vi "front pannel.vi"() -> ()   [LabVIEW 2013]
uses:
  XPS-C8 Controller/Examples/Global 1.vi
panel:
  out "KILL ALL ERROR":string
  in  "KILL ALL":bool
  out "error status 8":string
  out "error status 7":string
  out "error status 6":string
  out "error status 5":string
  out "error status 4":string
  out "error status 3":string
  out "error status 2":string
  out "error status 1":string
  out "position 8":dbl format="%#_13g"
  out "position 7":dbl format="%#_13g"
  out "position 6":dbl format="%#_13g"
  out "position 5":dbl format="%#_13g"
  out "position 4":dbl format="%#_13g"
  out "position 3":dbl format="%#_13g"
  out "position 2":dbl format="%#_13g"
  out "position 1":dbl format="%#_13g"
  in  "move 8":bool
  in  "move 7":bool
  in  "move 6":bool
  in  "move 5":bool
  in  "move 4":bool
  in  "move 3":bool
  in  "move 2":bool
  in  "move 1":bool
  out "8":bool
  out "7":bool
  out "6":bool
  out "5":bool
  out "4":bool
  out "3":bool
  out "2":bool
  out "error":bool
  out "hardware status 8":string
  out "hardware status 7":string
  out "hardware status 6":string
  out "hardware status 5":string
  out "hardware status 4":string
  out "hardware status 3":string
  out "hardware status 2":string
  out "hardware status 1":string
  out "motor name 8":string
  out "motor name 7":string
  out "motor name 6":string
  out "motor name 5":string
  out "motor name 4":string
  out "motor name 3":string
  out "motor name 2":string
  out "motor name 1":string
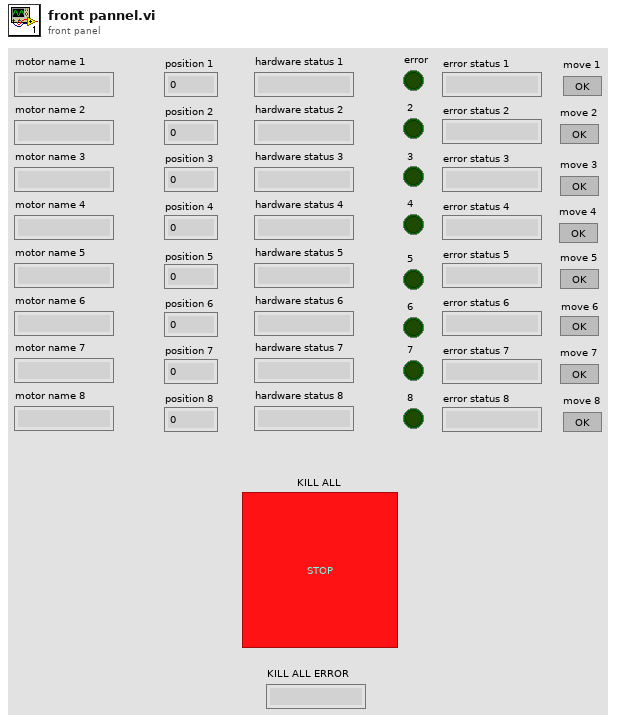
[diagram p1: front panel]
types:
  T1 = cluster{"connection TCP":refnum<k5>, "LogTo File":bool, "Log File refnum":refnum<file>, "no error if error log":bool}
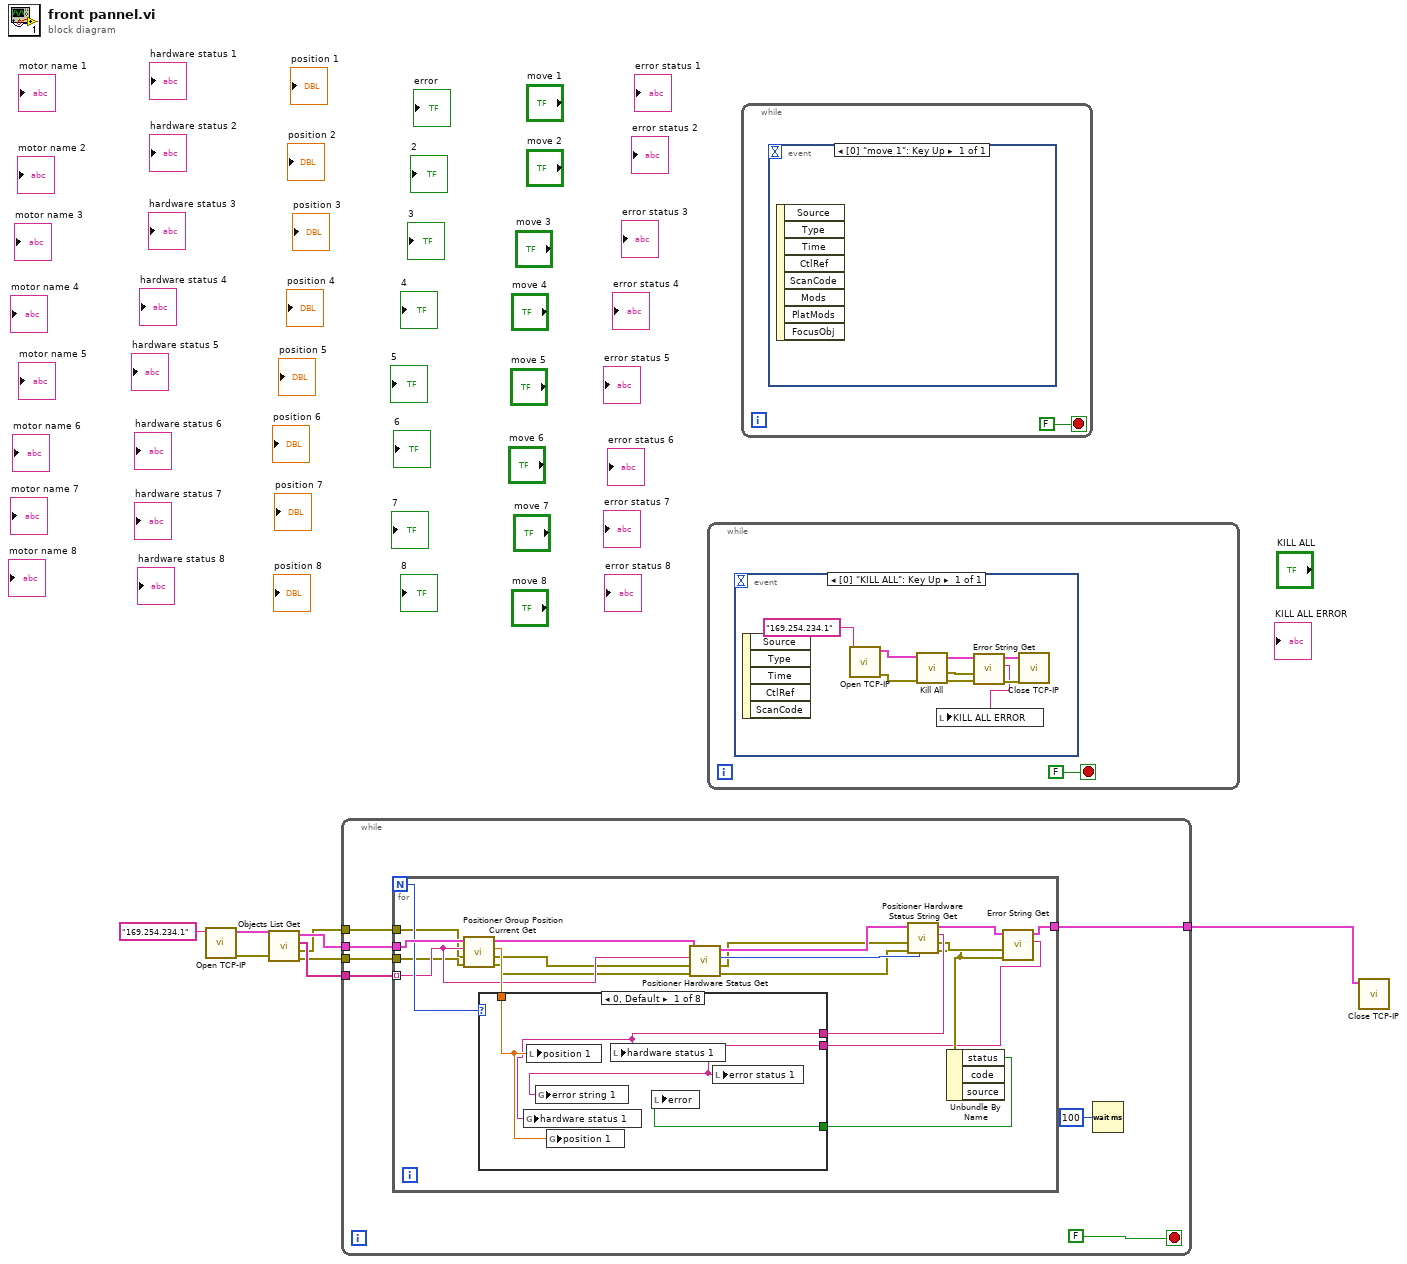
[diagram p0: block diagram]
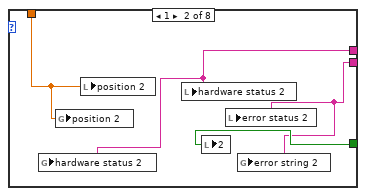
[diagram p2: hidden frame]
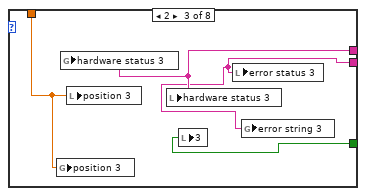
[diagram p3: hidden frame]
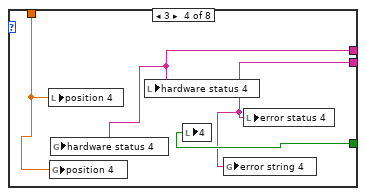
[diagram p4: hidden frame]
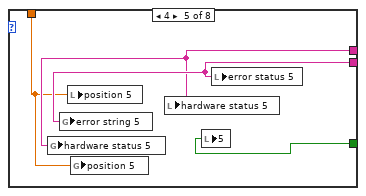
[diagram p5: hidden frame]
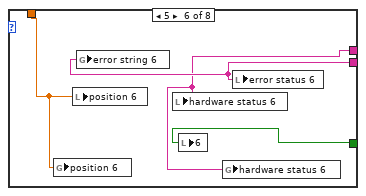
[diagram p6: hidden frame]
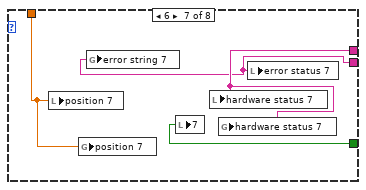
[diagram p7: hidden frame]
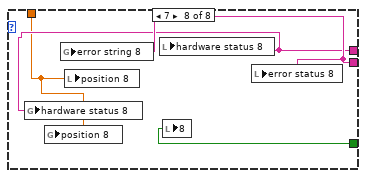
[diagram p8: hidden frame]
diagram:
  n1 = call <userlib>:"Open TCP-IP.vi"("IP address"="169.254.234.1") -> ("error out"=w3:errorcluster, "Connection ID"=w7:T1)  [unwired: 8 in, 1 out]
  n2 = call <userlib>:"Objects List Get.vi"("error in (no error)"=w3, "connection ID in"=w7) -> ("error out"=w2:errorcluster, "XPS error out"=w1:errorcluster, "Positioners"=w8:string[], "connection ID out"=w6:T1)  [unwired: 4 in, 2 out]
  n3 = while {
    tunnel: w8 -> [w15]
    tunnel: w6 -> [w14]
    tunnel: [w11] -> w5
    tunnel: w2 -> [w10]
    tunnel: w1 -> [w9]
    stop <- FALSE stop-if-true
    n4 = for {
      N -> [w31]
      tunnel: w15 -> [w28] mode=indexing
      tunnel: w14 -> [w35]
      tunnel: [w17] -> w11
      tunnel: w10 -> [w27]
      tunnel: w9 -> [w23]
      n5 = call "Positioner Group Position Current Get.vi"("error in (no error)"=w27, "XPS error in (no error)"=w23, "Positioner Name (250 c max)"=w28, "connection ID in"=w35) -> ("error out"=w26:errorcluster, "XPS error out"=w22:errorcluster, "Current position (units)"=w30:dbl, "connection ID out"=w34:T1)  [unwired: 4 in]
      n6 = call "Positioner Hardware Status Get.vi"("error in (no error)"=w26, "XPS error in (no error)"=w22, "Positioner Name (250 c max)"=w28, "connection ID in"=w34) -> ("error out"=w25:errorcluster, "XPS error out"=w21:errorcluster, "Positioner Hardware Status"=w32:i32, "connection ID out"=w33:T1)  [unwired: 4 in]
      n7 = call "Positioner Hardware Status String Get.vi"("Positioner Hardware Status"=w32, "error in (no error)"=w25, "XPS error in (no error)"=w21, "connection ID in"=w33) -> ("error out"=w19:errorcluster, "XPS error out"=w20:errorcluster, "Positioner Hardware Status String"=w29:string, "connection ID out"=w18:T1)  [unwired: 4 in]
      n8 = Unbundle By Name(w19) -> ("status"=w24:bool)  [unwired: 2 out]
      n9 = call "Error String Get.vi"("error in (no error)"=w19, "XPS error in"=w20, "connection ID in"=w18) -> ("Error String"=w16:string, "connection ID out"=w17:T1)  [unwired: 5 in, 2 out]
      n10 = case shown="0, Default" w31 {
        tunnel: w30 -> [w38 w40 w46 w50 w52 w56 w60 w64]
        tunnel: w29 -> [w36 w41 w45 w48 w53 w57 w62 w65]
        tunnel: w24 -> [w39 w43 w47 w51 w55 w59 w63 w67]
        tunnel: w16 -> [w37 w42 w44 w49 w54 w58 w61 w66]
        frame 0, Default {
          n11 = global write "Global 1.vi" "hardware status 1"(w36) -> ()
          n12 = local write "position 1"(w38) -> ()
          n13 = global write "Global 1.vi" "error string 1"(w37) -> ()
          n14 = global write "Global 1.vi" "position 1"(w38) -> ()
          n15 = local write "hardware status 1"(w36) -> ()
          n16 = local write "error"(w39) -> ()
          n17 = local write "error status 1"(w37) -> ()
        }
        frame 1 {
          n18 = global write "Global 1.vi" "hardware status 2"(w41) -> ()
          n19 = global write "Global 1.vi" "position 2"(w40) -> ()
          n20 = local write "position 2"(w40) -> ()
          n21 = local write "hardware status 2"(w41) -> ()
          n22 = local write "2"(w43) -> ()
          n23 = local write "error status 2"(w42) -> ()
          n24 = global write "Global 1.vi" "error string 2"(w42) -> ()
        }
        frame 2 {
          n25 = global write "Global 1.vi" "position 3"(w46) -> ()
          n26 = global write "Global 1.vi" "hardware status 3"(w45) -> ()
          n27 = local write "position 3"(w46) -> ()
          n28 = local write "hardware status 3"(w45) -> ()
          n29 = local write "3"(w47) -> ()
          n30 = local write "error status 3"(w44) -> ()
          n31 = global write "Global 1.vi" "error string 3"(w44) -> ()
        }
        frame 3 {
          n32 = local write "position 4"(w50) -> ()
          n33 = global write "Global 1.vi" "position 4"(w50) -> ()
          n34 = global write "Global 1.vi" "hardware status 4"(w48) -> ()
          n35 = local write "hardware status 4"(w48) -> ()
          n36 = local write "4"(w51) -> ()
          n37 = global write "Global 1.vi" "error string 4"(w49) -> ()
          n38 = local write "error status 4"(w49) -> ()
        }
        frame 4 {
          n39 = global write "Global 1.vi" "hardware status 5"(w53) -> ()
          n40 = global write "Global 1.vi" "error string 5"(w54) -> ()
          n41 = local write "position 5"(w52) -> ()
          n42 = global write "Global 1.vi" "position 5"(w52) -> ()
          n43 = local write "hardware status 5"(w53) -> ()
          n44 = local write "5"(w55) -> ()
          n45 = local write "error status 5"(w54) -> ()
        }
        frame 5 {
          n46 = global write "Global 1.vi" "position 6"(w56) -> ()
          n47 = local write "position 6"(w56) -> ()
          n48 = global write "Global 1.vi" "error string 6"(w58) -> ()
          n49 = local write "hardware status 6"(w57) -> ()
          n50 = local write "6"(w59) -> ()
          n51 = global write "Global 1.vi" "hardware status 6"(w57) -> ()
          n52 = local write "error status 6"(w58) -> ()
        }
        frame 6 {
          n53 = local write "position 7"(w60) -> ()
          n54 = global write "Global 1.vi" "position 7"(w60) -> ()
          n55 = global write "Global 1.vi" "error string 7"(w61) -> ()
          n56 = local write "7"(w63) -> ()
          n57 = local write "hardware status 7"(w62) -> ()
          n58 = global write "Global 1.vi" "hardware status 7"(w62) -> ()
          n59 = local write "error status 7"(w61) -> ()
        }
        frame 7 {
          n60 = global write "Global 1.vi" "hardware status 8"(w65) -> ()
          n61 = global write "Global 1.vi" "position 8"(w64) -> ()
          n62 = global write "Global 1.vi" "error string 8"(w66) -> ()
          n63 = local write "position 8"(w64) -> ()
          n64 = local write "hardware status 8"(w65) -> ()
          n65 = local write "8"(w67) -> ()
          n66 = local write "error status 8"(w66) -> ()
        }
      }
    }
    n67 = Wait (ms)(milliseconds to wait=u32 100) -> ()  [unwired: 1 out]
  }
  n68 = while {
    stop <- FALSE stop-if-true
    n69 = event shown="[0] \"KILL ALL\": Key Up" {
      selector: _ -> [_]
      dyn-events: _ -> [_]
      timeout: _ -> [_]
      event "KILL ALL": Key Up {
        n70 = event-data() -> ()  [unwired: 1 in, 5 out]
        n71 = call <userlib>:"Open TCP-IP.vi"("IP address"="169.254.234.1") -> ("error out"=w76:errorcluster, "Connection ID"=w77:T1)  [unwired: 8 in, 1 out]
        n72 = call "Kill All.vi"("error in (no error)"=w76, "connection ID in"=w77) -> ("error out"=w74:errorcluster, "XPS error out"=w75:errorcluster, "connection ID out"=w71:T1)  [unwired: 7 in]
        n73 = call "Error String Get.vi"("error in (no error)"=w74, "XPS error in"=w75, "connection ID in"=w71) -> ("error out"=w73:errorcluster, "Error String"=w70:string, "connection ID out"=w72:T1)  [unwired: 5 in, 1 out]
        n74 = local write "KILL ALL ERROR"(w70) -> ()
        n75 = call <userlib>:"Close TCP-IP.vi"("error in (no error)"=w73, "connection ID in"=w72) -> ()  [unwired: 9 in, 1 out]
      }
    }
  }
  n76 = while {
    stop <- FALSE stop-if-true
    n77 = event shown="[0] \"move 1\": Key Up" {
      selector: _ -> [_]
      dyn-events: _ -> [_]
      timeout: _ -> [_]
      event "move 1": Key Up {
        n78 = event-data() -> ()  [unwired: 1 in, 8 out]
      }
    }
  }
  n79 = call <userlib>:"Close TCP-IP.vi"("connection ID in"=w5) -> ()  [unwired: 10 in, 1 out]
